vi "Cron Next (Unix-compatible).vi"(9 "Nb Occurences (min: 1)":u16=1 min=1, 10 "Reference timestamp (Now)":timestamp, 11 "Cron Expression":string="* * * ? *") -> (1 "Occurences":timestamp[](array[timestamp]), 2 "Next Occurence":timestamp, 3 "syntax valid?":bool)   [LabVIEW 2013, in "openCron.lvlib"]
uses:
  openCron.lvlib
  Cron.Unix/Cron.Unix.lvclass
  Cron/Cron.lvclass
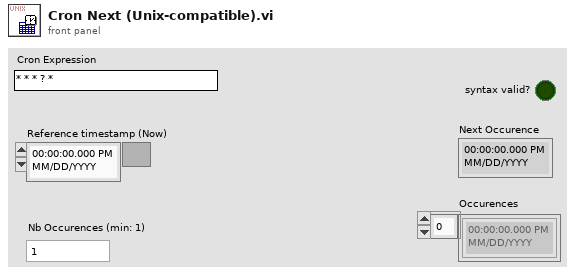
[diagram p1: front panel]
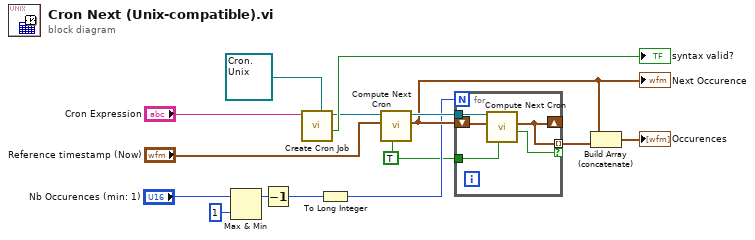
[diagram p0: block diagram]
diagram:
  w2 = TRUE ("Ignore DST?")
  n1 = Max & Min(x="Nb Occurences (min: 1)", y=u16 1) -> (max(x,y)=w8:u16)  [unwired: 1 out]
  n2 = Decrement(x=w8) -> (x-1=w7:u16)
  n3 = call "Create Cron Job.vi"("Cron in"=refnum<class "Cron.Unix.lvclass"> refnum ("openCron.lvlib:Cron.Unix.lvclass"), "Cron Expression"="Cron Expression") -> ("expression valid"=→"syntax valid?":bool, "Cron out"=w13:refnum<class "Cron.Unix.lvclass">)  [unwired: 7 in, 1 out]
  n4 = To Long Integer(number=w7) -> (32bit integer=w3:i32)
  n5 = call "Compute Next Cron.vi"("Ignore DST?"=w2, "Time Stamp (Now)"="Reference timestamp (Now)", "Cron in"=w13) -> ("Next Occurence"=w5:timestamp, "Cron out"=w11:refnum<class "Cron.Unix.lvclass">)  [unwired: 5 in, 2 out]
  "Next Occurence" <- w5
  n6 = for {
    N: w3 -> [_]
    shift-right: [w18] -> _
    shift-left: w5 -> [w20]
    tunnel: w11 -> [w19]
    tunnel: [w18] -> w6 mode=indexing if=w16
    tunnel: w2 -> [w17]
    n7 = call "Compute Next Cron.vi"("Ignore DST?"=w17, "Time Stamp (Now)"=w20, "Cron in"=w19) -> ("Occurence found"=w16:bool, "Next Occurence"=w18:timestamp)  [unwired: 5 in, 2 out]
  }
  n8 = Build Array (concatenate)(w5, w6) -> (→"Occurences":timestamp[])
